vi "MVE Import.vi"(11 "Full Path":string) -> (0 "error out":errorcluster, 3 "cancelled":bool)   [LabVIEW 2016]
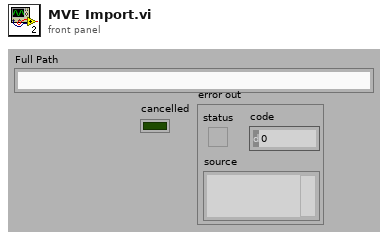
[diagram p1: front panel]
types:
  T1 = typedef "SCT Default Types.ctl" = cluster{"names":string[], "TDs":T2[]}
  T2 = typedef "NI_Variable.lvlib/Type Descriptor.ctl" = cluster{"Variant":variant}
  T3 = typedef "SCT Variable.ctl" = cluster{"Name":string, "TypeDesc":T2, "Type":string, "typedefs":string, "Attribs":T4, "FeaturePacks":string[], "Source":string}
  T4 = typedef "NI_Variable.lvlib/Attribs.ctl" = cluster{"Attrib":string, "Value":string}[]
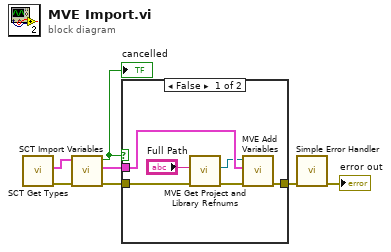
[diagram p0: block diagram]
diagram:
  n1 = call <resource>:"SCT Get Types.vi"() -> ("error out"=w6:errorcluster, "default types"=w7:T1)  [unwired: 9 in, 1 out]
  n2 = call <resource>:"SCT Import Variables.vi"("error in (no error)"=w6, "default types"=w7) -> ("error out"=w4:errorcluster, "Array"=w5:T3[], "Cancelled"=w3:bool)  [unwired: 7 in]
  "cancelled" <- w3
  n3 = case shown="False" w3 {
    tunnel: w5 -> [w9 _]
    tunnel: w4 -> [w12 w14]
    tunnel: [w10 w14] -> w2
    frame False {
      n4 = call <resource>:"MVE Get Project and Library Refnums.vi"("error in (no error)"=w12, "Full Path"="Full Path") -> ("error out"=w11:errorcluster, "ProjectItem Refnum"=w8:refnum<vi>)  [unwired: 7 in, 1 out]
      n5 = call <resource>:"MVE Add Variables.vi"("error in (no error)"=w11, "variables"=w9, "ProjectItem Refnum"=w8) -> ("error out"=w10:errorcluster)  [unwired: 7 in, 1 out]
    }
    frame True {
    }
  }
  n6 = call <vilib>:"Simple Error Handler.vi"("error in (no error)"=w2) -> ("error out"=→"error out":errorcluster)  [unwired: 4 in, 4 out]
